vi "HEWH Update Last Terminate Condition.vi"(8 "error in":errorcluster, 10 "Terminate Condition":T3, 11 "PRAT/RLT Sequence":T1[](array[typedef]) {"Time" format="%<%H:%M:%S>t"}) -> (0 "error out":errorcluster, 3 "PRAT/RLT Sequence (Output)":T1[](array[typedef]) {"Time" format="%<%H:%M:%S>t"})   [LabVIEW 2023]
uses:
  Type Definitions/PRAT Test.ctl
  Utility/Save File/File Setup (Public)/Type Definition/Save File HEWH Heating Control Mode.ctl
  Draw Water Specific/Type Definitions/Terminate Draw Conditions.ctl
  Type Definitions/HEWH Start Conditions.ctl
  Draw Water Specific/Type Definitions/Check Special Condtions.ctl
  Draw Water Specific/Type Definitions/HEWH Special Condition Check.ctl
  Type Definitions/HEWH Draw Flag ENUM.ctl
  Utility/Save File/File Setup.lvlib
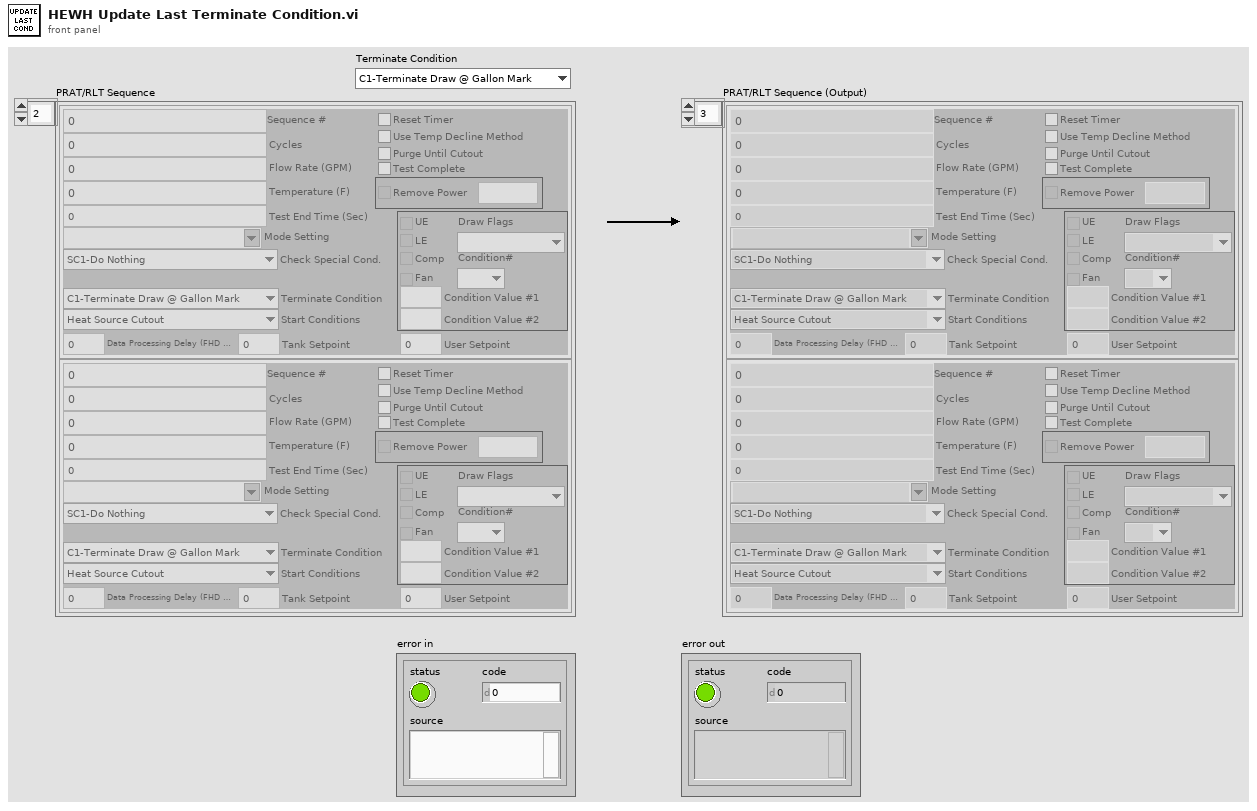
[diagram p1: front panel]
types:
  T1 = typedef "PRAT Test.ctl" = cluster{"Sequence #":dbl, "Cycles":i32, "Mode Setting":T2, "Flow Rate (GPM)":dbl, "Temperature (F)":dbl, "Reset Timer":bool, "Use Temp Decline Method":bool, "Terminate Condition":T3, "Condition Value #1":dbl, "UE":bool, "LE":bool, "Comp":bool, "Fan":bool, "Test End Time (Sec)":dbl, "Purge Until Cutout":bool, "Start Conditions":T4, "Condition Value #2":dbl, "Remove Power":bool, "Time":dbl, "Check Special Cond.":T5, "Condition#":T6, "Draw Flags":T7, "Data Processing Delay (FHD 15sec, UEF 5 Sec)":dbl, "Test Complete":bool, "User Setpoint":dbl, "Tank Setpoint":dbl}
  T2 = typedef "File Setup.lvlib/Save File HEWH Heating Control Mode.ctl" = string
  T3 = typedef "Terminate Draw Conditions.ctl" = enum16{"C1-Terminate Draw @ Gallon Mark", "C2-Special Last Draw (HU Test)", "C3-RTD Out <=", "C4-Mean Tank Temp <=", "C5-Decrease RTD Out (Deg F)", "C6-Time (Seconds)", "C7-Until Any Heat Source", "C8-Specific Heat Source", "C9-Do Nothing", "C10-Inlet Outlet RTD Temp Delta"}
  T4 = typedef "HEWH Start Conditions.ctl" = enum16{"Heat Source Cutout", "At Time (Seconds)", "Every X (Seconds)", "T2 >= X° Below Setpoint", "Seconds From Complete", "Wait for LE & Comp Cutout", "Wait for Comp Cutout", "Wait for LE Cutout", "Wait for UE Cutout", "Start Immediately"}
  T5 = typedef "Check Special Condtions.ctl" = enum16{"SC1-Do Nothing", "SC2-Check Heat Source (On-C2/Off-C1)", "SC3-Check Skip Condition", "SC4-Check Heat Source ON/Fail", "SC5-Keep Draw Valves Open", "SC6-Skip Purge"}
  T6 = typedef "HEWH Special Condition Check.ctl" = enum16{"N/A", "C1", "C2", "Reset/Fail", "Skip Draw Sequence"}
  T7 = typedef "HEWH Draw Flag ENUM.ctl" = enum16{"N/A", "None(0)", "Sml(1)", "Med(2)", "SmlMed(3)", "Lrg(4)", "SmlLrg(5)", "MedLrg(6)", "SmlMedLrg(7)"}
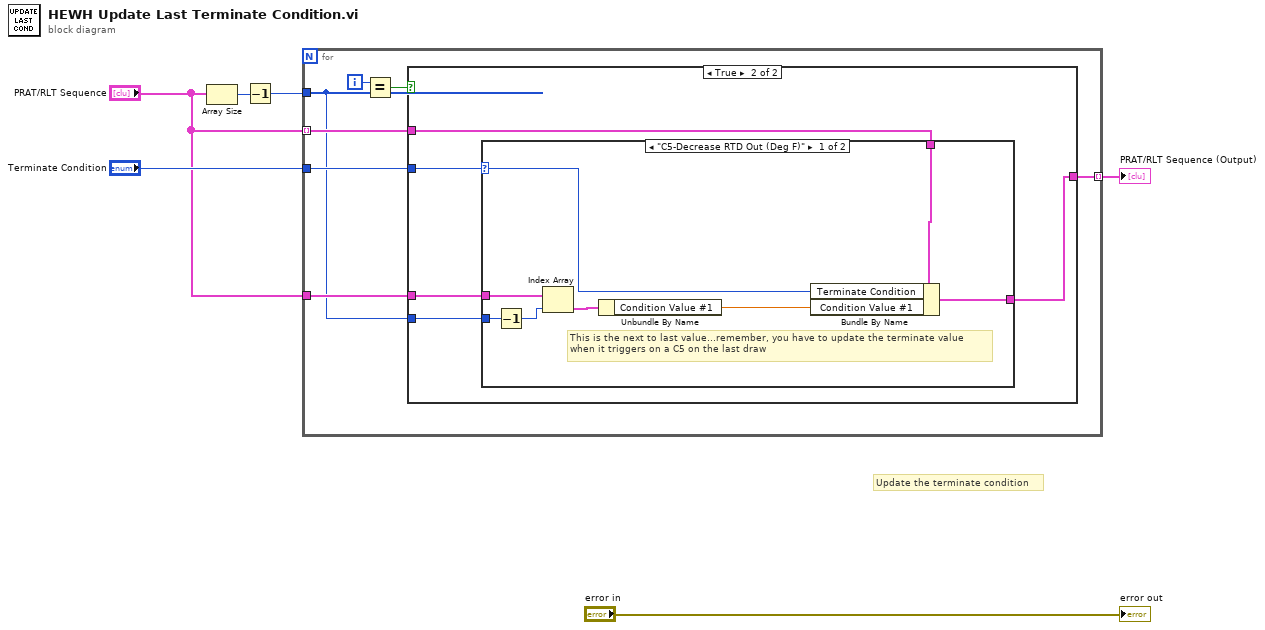
[diagram p0: block diagram]
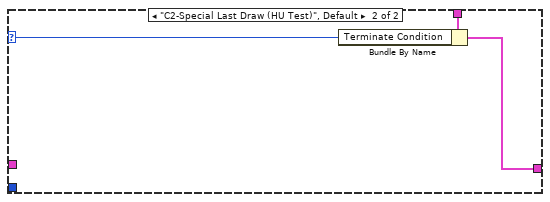
[diagram p3: hidden frame]
diagram:
  # "Update the terminate condition"
  n1 = Array Size(array="PRAT/RLT Sequence") -> (size(s)=w5:i32)
  n2 = Decrement(x=w5) -> (x-1=w3:i32)
  n3 = for {
    tunnel: "PRAT/RLT Sequence" -> [w11] mode=indexing
    tunnel: w3 -> [w7]
    tunnel: [w10] -> w6 mode=indexing
    tunnel: "Terminate Condition" -> [w9]
    tunnel: "PRAT/RLT Sequence" -> [w8]
    i -> [w13]
    n4 = Equal?(x=w13, y=w7) -> (x = y?=w12:bool)
    n5 = case shown="True" w12 {
      tunnel: w11 -> [w14 w19]
      tunnel: [w14 w17] -> w10
      tunnel: w9 -> [_ w18]
      tunnel: w8 -> [_ w16]
      tunnel: w7 -> [_ w15]
      frame False {
      }
      frame True {
        n6 = case shown="\"C5-Decrease RTD Out (Deg F)\"" w18 {
          selector: w18 -> [w20 w28]
          tunnel: w15 -> [w27 _]
          tunnel: w16 -> [w26 _]
          tunnel: w19 -> [w23 w30]
          tunnel: [w22 w29] -> w17
          frame "C5-Decrease RTD Out (Deg F)" {
            # "This is the next to last value...remember, you have to update the terminate value\nwhen it triggers on a C5 on the last draw"
            n7 = Decrement(x=w27) -> (x-1=w25:i32)
            n8 = Index Array(array=w26, index=w25) -> (element=w24:T1)
            n9 = Unbundle By Name(w24) -> ("Condition Value #1"=w21:dbl)
            n10 = Bundle By Name(cluster=w23, "Terminate Condition"=w20, "Condition Value #1"=w21) -> (w22:T1)
          }
          frame "C2-Special Last Draw (HU Test)", Default {
            n11 = Bundle By Name(cluster=w30, "Terminate Condition"=w28) -> (w29:T1)
          }
        }
      }
    }
  }
  "PRAT/RLT Sequence (Output)" <- w6
  "error out" <- "error in"
